vi "Execution_Appli_SetupSpecificSettings.vi"(8 "error in":errorcluster, 11 "EVE_AppSpecific in":refnum<class "EVE_AppSpecific.lvclass">) -> (0 "error out":errorcluster, 3 "EVE_AppSpecific out":refnum<class "EVE_AppSpecific.lvclass">)   [LabVIEW 2013, in "EVE_AppSpecific.lvclass"]
uses:
  EVE_AppSpecific.lvclass
  EVE_AppSpecific.lvclass/EVE_AppSpecific.ctl
  EVE.lvclass
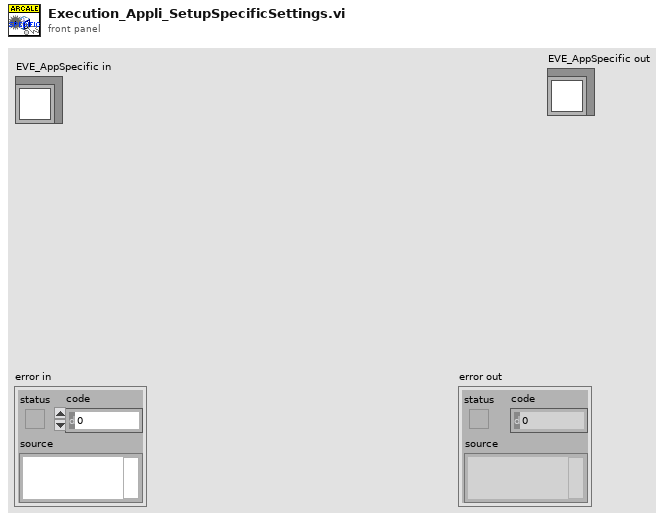
[diagram p1: front panel]
types:
  T1 = enum16{"open", "replace", "create", "open or create", "replace or create", "replace or create with confirmation"}
  T2 = typedef "EVE.lvclass/App_GenericSettings.ctl" = cluster{"SpecificSettings":cluster{"FolderPath":path, "XMLFile":string}, "Log":cluster{"MaxLogFiles":i32, "MaxLogMessagesPerFile":i32}, "Debug":cluster{"Active":bool}, "Dictionnary":cluster{"FolderPath":path, "TradFile":string}, "Ressources":cluster{"FolderPath":path}}
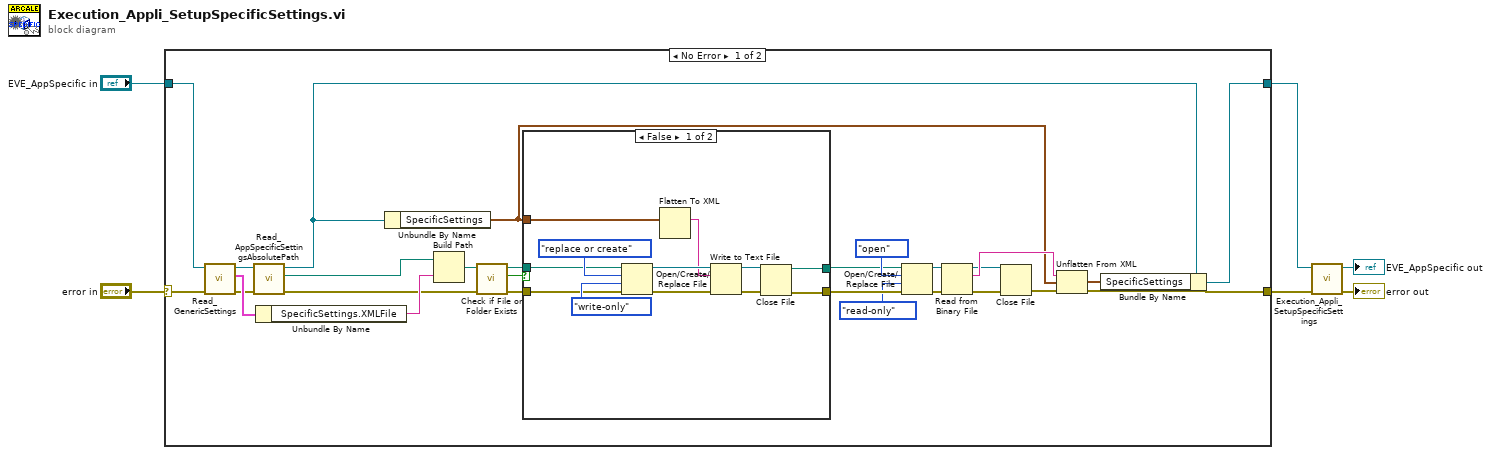
[diagram p0: block diagram]
diagram:
  n1 = case shown="No Error" "error in" {
    selector: "error in" -> [w28 w49]
    tunnel: [w7 w49] -> w3
    tunnel: [w10 w48] -> w2
    tunnel: "EVE_AppSpecific in" -> [w23 w48]
    frame No Error {
      n2 = call-dynamic "Read_GenericSettings.vi"("error in (no error)"=w28, "EVE in"=w23) -> ("error out"=w25:errorcluster, "GenericSettings"=w29:T2, "EVE out"=w26:refnum<class "EVE_AppSpecific.lvclass">)  [unwired: 7 in]
      n3 = call-dynamic "Read_AppSpecificSettingsAbsolutePath.vi"("error in (no error)"=w25, "EVE in"=w26) -> ("error out"=w24:errorcluster, "AppSpecificSettingsAbsolutePath"=w27:path, "EVE out"=w11:refnum<class "EVE_AppSpecific.lvclass">)  [unwired: 7 in]
      n4 = Unbundle By Name(w29) -> ("SpecificSettings.XMLFile"=w32:string)
      n5 = Unbundle By Name(w11) -> ("SpecificSettings"=w12:cluster{"Numeric":dbl})
      n6 = Build Path(base path=w27, name or relative path=w32) -> (appended path=w33:path)
      n7 = call <vilib>:"Check if File or Folder Exists.vi"("error in (no error)"=w24, "path"=w33) -> ("error out"=w30:errorcluster, "file or folder exists?"=w31:bool, "dup path"=w22:path)  [unwired: 7 in]
      n8 = case shown="False" w31 {
        tunnel: w30 -> [w37 w47]
        tunnel: [w35 w47] -> w15
        tunnel: w22 -> [w38 w46]
        tunnel: w12 -> [w45 _]
        tunnel: [w34 w46] -> w14
        frame False {
          n9 = Open/Create/Replace File(file path (use dialog)=w38, error in=w37, operation (0:open)=T1."replace or create", access (0:read/write)=enum16{"read/write", "read-only", "write-only"}."write-only") -> (refnum out=w41:refnum<file>, error out=w42:errorcluster)  [unwired: 2 in, 1 out]
          n10 = Flatten To XML(anything=w45) -> (xml string=w36:string)
          n11 = Write to Text File(file (use dialog)=w41, text=w36, error in=w42) -> (refnum out=w39:refnum<file>, error out=w40:errorcluster)  [unwired: 1 in, 1 out]
          n12 = Close File(refnum=w39, error in=w40) -> (path=w34:path, error out=w35:errorcluster)
        }
        frame True {
        }
      }
      n13 = Open/Create/Replace File(file path (use dialog)=w14, error in=w15, operation (0:open)=T1."open", access (0:read/write)=enum16{"read/write", "read-only", "write-only"}."read-only") -> (refnum out=w17:refnum<file>, error out=w19:errorcluster)  [unwired: 2 in, 1 out]
      n14 = Read from Binary File(8:w19, 11:w17) -> (0:w20:errorcluster, 2:w21:string, 3:w18:refnum<file>)  [unwired: 4 in, 1 out]
      n15 = Close File(refnum=w18, error in=w20) -> (error out=w8:errorcluster)  [unwired: 1 out]
      n16 = Unflatten From XML(xml string=w21, type=w12, error in (no error)=w8) -> (value=w9:cluster{"Numeric":dbl}, error out=w7:errorcluster)
      n17 = Bundle By Name(cluster=w11, "SpecificSettings"=w9) -> (w10:refnum<class "EVE_AppSpecific.lvclass">)
    }
    frame Error {
    }
  }
  n18 = call-parent "Execution_Appli_SetupSpecificSettings.vi"("error in"=w3, "EVE in"=w2) -> ("error out"=→"error out":errorcluster, "EVE out"=→"EVE_AppSpecific out":refnum<class "EVE_AppSpecific.lvclass">)  [unwired: 8 in]
